vi "Customize Droplets Graph.vi"(6 "DropletDBListBoxCtl":T1, 7 "Array of Graphs":cluster{"Ramp Pattern":dbl[], dbl[]}[](array[cluster]), 8 "error in (no error)":errorcluster, 9 "Normalized number of Droplets vs. Temperature 2":cluster{"Ramp Pattern":dbl[], dbl[]}(graph), 10 "Inlcude Total in Graph":bool, 11 "Graph":refnum<vi>) -> (0 "error out":errorcluster, 3 "Normalized number of Droplets vs. Temperature":cluster{"Ramp Pattern":dbl[], dbl[]}[](graph))   [LabVIEW 2013]
doc: "Use this template to build a VI to use as a subVI."
uses:
  TypeDef/DropletDBListBox.ctl
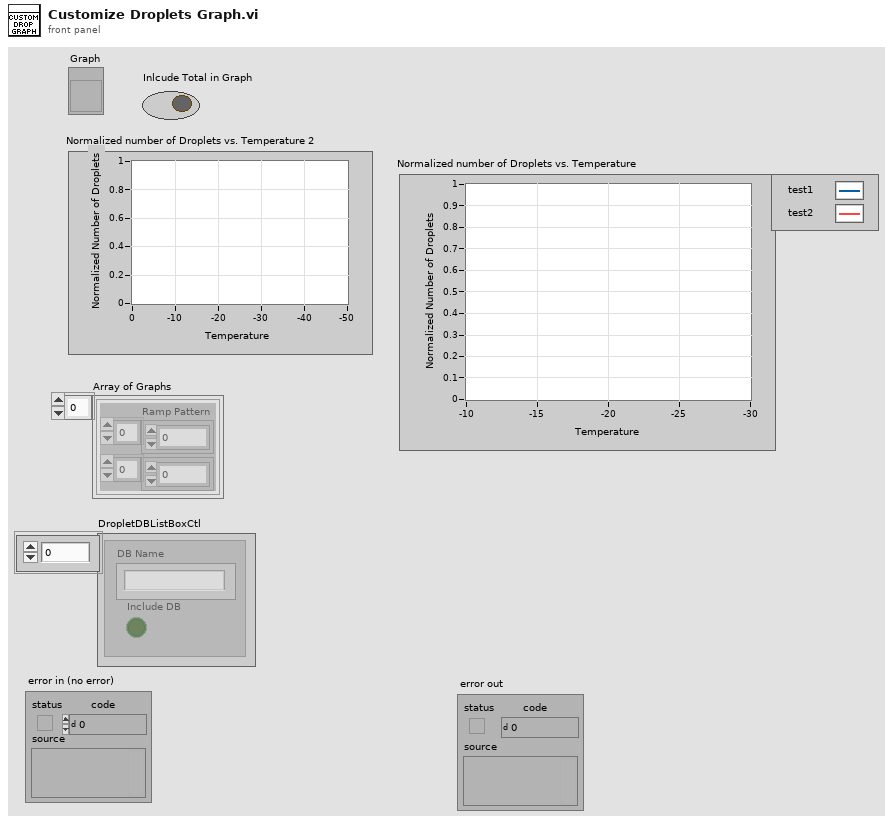
[diagram p1: front panel]
types:
  T1 = typedef "DropletDBListBox.ctl" = cluster{"DB Name":string, "Include DB":bool}[]
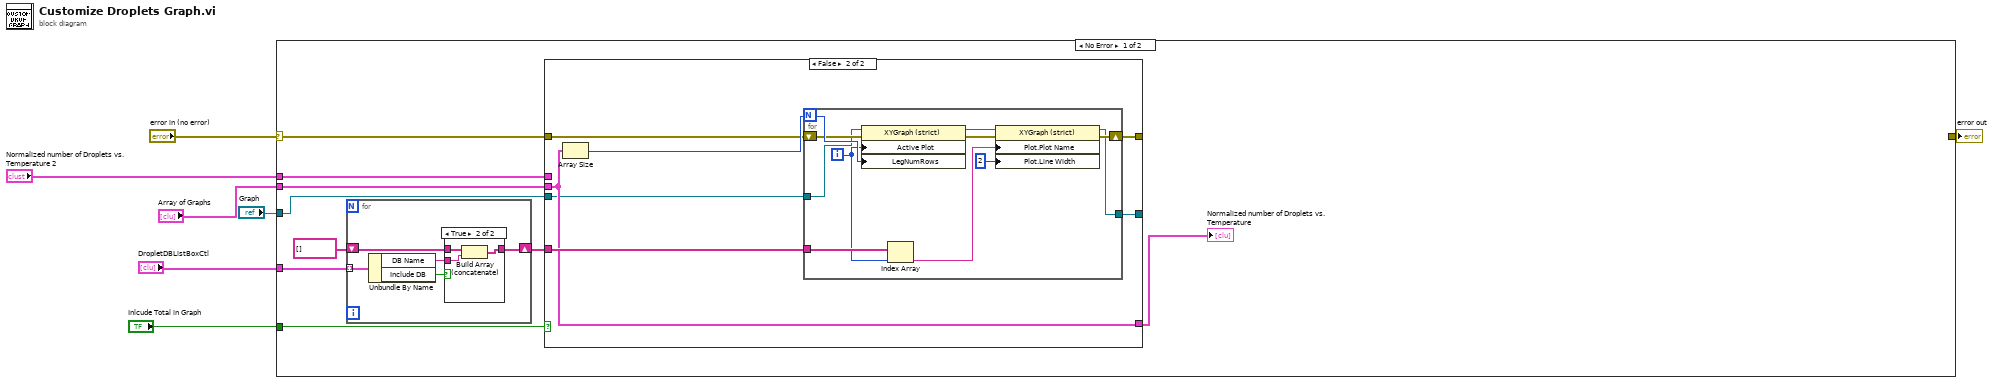
[diagram p0: block diagram]
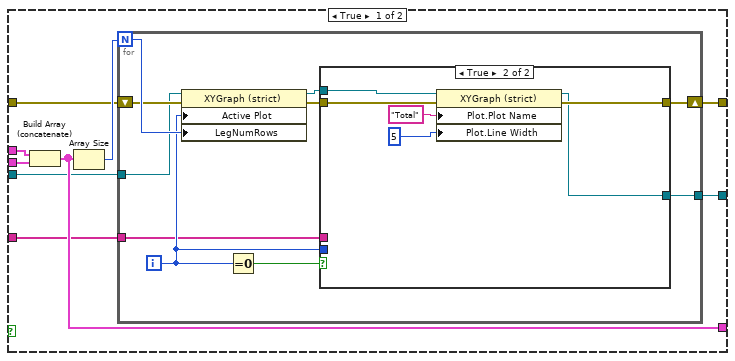
[diagram p3: hidden frame]
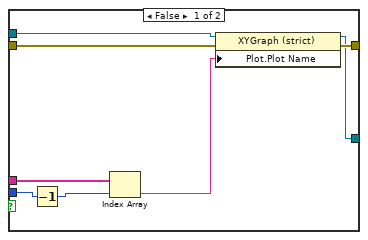
[diagram p4: hidden frame]
diagram:
  n1 = case shown="No Error" "error in (no error)" {
    selector: "error in (no error)" -> [w11 w77]
    tunnel: [_ w77] -> w6
    tunnel: "Inlcude Total in Graph" -> [w15 _]
    tunnel: "DropletDBListBoxCtl" -> [w13 _]
    tunnel: "Array of Graphs" -> [w8 _]
    tunnel: "Normalized number of Droplets vs. Temperature 2" -> [w12 _]
    tunnel: "Graph" -> [w10 _]
    frame No Error {
      n2 = for {
        tunnel: w13 -> [w21] mode=indexing
        shift-right: [w18] -> w16
        shift-left: string[] [] -> [w17]
        n3 = Unbundle By Name(w21) -> ("DB Name"=w19:string, "Include DB"=w20:bool)
        n4 = case shown="True" w20 {
          tunnel: w19 -> [_ w25]
          tunnel: [w22 w24] -> w18
          tunnel: w17 -> [w22 w23]
          frame False {
          }
          frame True {
            n5 = Build Array (concatenate)(w23, w25) -> (w24:string[])
          }
        }
      }
      n6 = case shown="False" w15 {
        tunnel: w12 -> [w34 _]
        tunnel: w8 -> [w33 w63]
        tunnel: [w31 w63] -> w9
        tunnel: w16 -> [w30 w64]
        tunnel: w11 -> [w29 w62]
        tunnel: [w28 w61] -> _
        tunnel: w10 -> [w27 w60]
        tunnel: [w26 w59] -> _
        frame True {
          n7 = Build Array (concatenate)(w34, w33) -> (w31:cluster{"Ramp Pattern":dbl[], dbl[]}[])
          n8 = Array Size(array=w31) -> (size(s)=w32:i32)
          n9 = for {
            N: w32 -> [w43]
            tunnel: w30 -> [w40]
            shift-right: [w38] -> w28
            shift-left: w29 -> [w39]
            tunnel: w27 -> [w37]
            tunnel: [w35] -> w26
            i -> [w41]
            n10 = property on="Property Node" class="XYGraph (strict)"(reference=w37, error in=w39, "Active Plot"=w41, "LegNumRows"=w43) -> (reference out=w36:refnum<vi>, error out=w44:errorcluster)
            n11 = Equal To 0?(x=w41) -> (x = 0?=w42:bool)
            n12 = case shown="True" w42 {
              tunnel: w44 -> [w48 w58]
              tunnel: w41 -> [w52 _]
              tunnel: w40 -> [w50 _]
              tunnel: [w47 w55] -> w38
              tunnel: w36 -> [w46 w54]
              tunnel: [w45 w53] -> w35
              frame False {
                n13 = Decrement(x=w52) -> (x-1=w51:i32)
                n14 = Index Array(array=w50, index=w51) -> (element=w49:string)
                n15 = property on="Property Node" class="XYGraph (strict)"(reference=w46, error in=w48, "Plot.Plot Name"=w49) -> (reference out=w45:refnum<vi>, error out=w47:errorcluster)
              }
              frame True {
                n16 = property on="Property Node" class="XYGraph (strict)"(reference=w54, error in=w58, "Plot.Plot Name"="Total", "Plot.Line Width"=u8 5) -> (reference out=w53:refnum<vi>, error out=w55:errorcluster)
              }
            }
          }
        }
        frame False {
          n17 = Array Size(array=w63) -> (size(s)=w65:i32)
          n18 = for {
            N: w65 -> [w76]
            tunnel: w64 -> [w75]
            shift-right: [w69] -> w61
            shift-left: w62 -> [w70]
            tunnel: w60 -> [w68]
            tunnel: [w66] -> w59
            i -> [w73]
            n19 = property on="Property Node" class="XYGraph (strict)"(reference=w68, error in=w70, "Active Plot"=w73, "LegNumRows"=w76) -> (reference out=w67:refnum<vi>, error out=w71:errorcluster)
            n20 = Index Array(array=w75, index=w73) -> (element=w74:string)
            n21 = property on="Property Node" class="XYGraph (strict)"(reference=w67, error in=w71, "Plot.Plot Name"=w74, "Plot.Line Width"=u8 2) -> (reference out=w66:refnum<vi>, error out=w69:errorcluster)
          }
        }
      }
      "Normalized number of Droplets vs. Temperature" <- w9
    }
    frame Error {
    }
  }
  "error out" <- w6
